vi "Send Remote Reply.vi"(7 "Original Payload":T1, 8 "error in (no error)":errorcluster, 9 "Message Type":string, 10 "Message":refnum<class "Message.lvclass">, 11 "VolatusAPI in":refnum<class "VolatusAPI.lvclass">) -> (0 "error out":errorcluster, 3 "VolatusAPI out":refnum<class "VolatusAPI.lvclass">)   [LabVIEW 2020, in "Volatus.lvlib" / "VolatusAPI.lvclass"]
uses:
  VolatusAPI.lvclass
  VolatusAPI.lvclass/VolatusAPI.ctl
  lv-vecto/Vecto/TCPMessageService/TCPMessageAPI.lvclass
  lv-protoc/LV-Proto/Message/Message.lvclass
  lv-vecto/Vecto/proto/TcpPayload/Data.ctl
  lv-vecto/Vecto/proto/TcpPayload/TcpPayload.lvlib
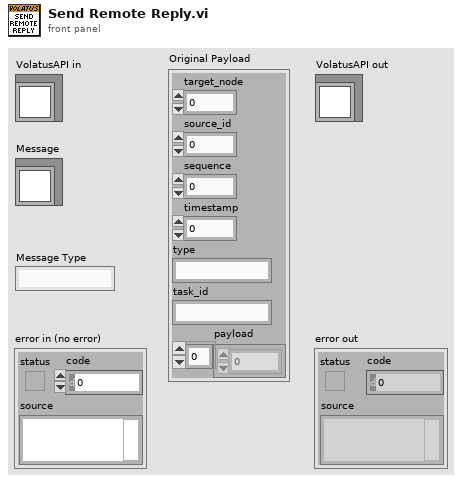
[diagram p1: front panel]
types:
  T1 = typedef "TcpPayload.lvlib/Data.ctl" = cluster{"target_node":u32, "source_id":u32, "sequence":u32, "timestamp":u64, "type":string, "task_id":string, "payload":u8[]}
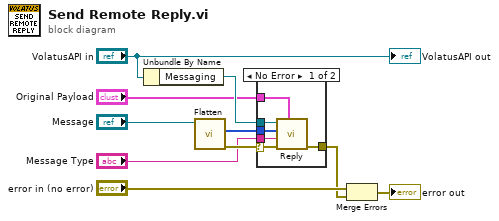
[diagram p0: block diagram]
diagram:
  n1 = Unbundle By Name("VolatusAPI in") -> ("Messaging"=w8:refnum<class "TCPMessageAPI.lvclass">)
  n2 = call-dynamic "Flatten.vi"("Message in"="Message") -> ("error out"=w4:errorcluster, "Buffer"=w5:u8[])  [unwired: 8 in, 1 out]
  n3 = case shown="No Error" w4 {
    selector: w4 -> [w13 w17]
    tunnel: w8 -> [w16 _]
    tunnel: "Original Payload" -> [w15 _]
    tunnel: w5 -> [w14 _]
    tunnel: "Message Type" -> [w12 _]
    tunnel: [w11 w17] -> w1
    frame No Error {
      n4 = call "Reply.vi"("Original Payload"=w15, "error in (no error)"=w13, "Type"=w12, "Payload"=w14, "TCPMessageAPI in"=w16) -> ("error out"=w11:errorcluster)  [unwired: 5 in, 1 out]
    }
    frame Error {
    }
  }
  n5 = Merge Errors("error in (no error)", w1) -> (→"error out":errorcluster)
  "VolatusAPI out" <- "VolatusAPI in"
